vi "test.vi"() -> ()   [LabVIEW 2016, in "TCP文件传输系统.lvlib"]
uses:
  <vilib>/Utility/error.llb/whitespace.ctl
  <vilib>/Utility/sysdir.llb/System Directory Type.ctl
panel:
  out "枚举":T1(ring)
  in  "Version":string="版本升级文档.txt"
  out "TCP发送全局簇":T2
  out "文件传输的路径":path
  in  "Application":string="平台数据传输系统.exe"
  in  "远程端口或服务名称":u16=11234
  out "本机网络地址":string="192.168.1.250"
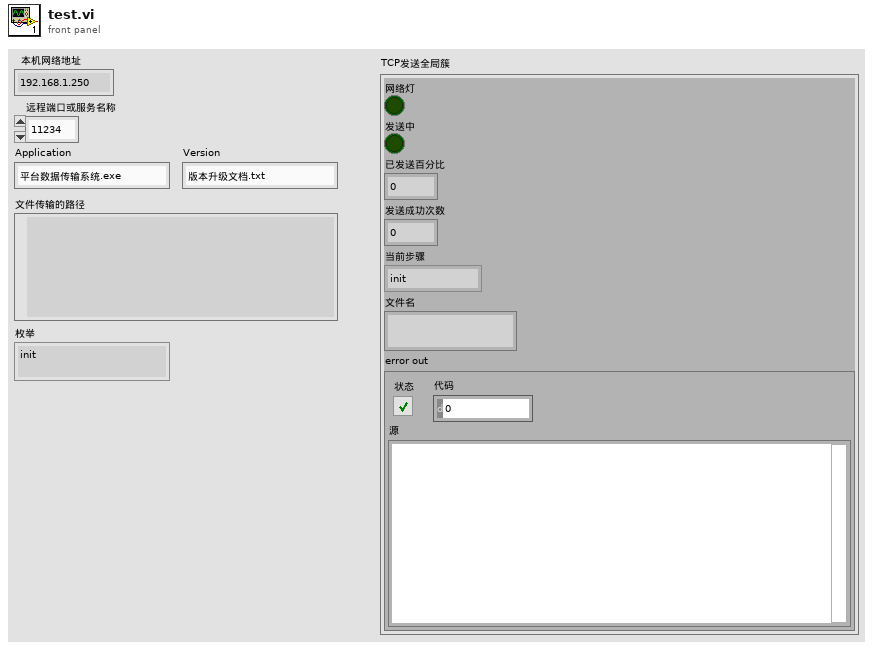
[diagram p1: front panel]
types:
  T1 = enum16{"init", "send version", "send version end", "send application", "send application end", "over"}
  T2 = cluster{"网络灯":bool, "发送中":bool, "已发送百分比":u8, "发送成功次数":dbl, "当前步骤":enum16{"init", "sendhead", "sendcontent", "sendsuccess", "over"}, "文件名":string, "error out":errorcluster}
  T3 = enum16{"Standard", "Buffered", "CRLF", "Immediate"}
  T4 = enum32{"Bad", "Idle", "Run top level", "Running"}
  T5 = typedef "whitespace.ctl" = u16
  T6 = typedef "System Directory Type.ctl" = i32
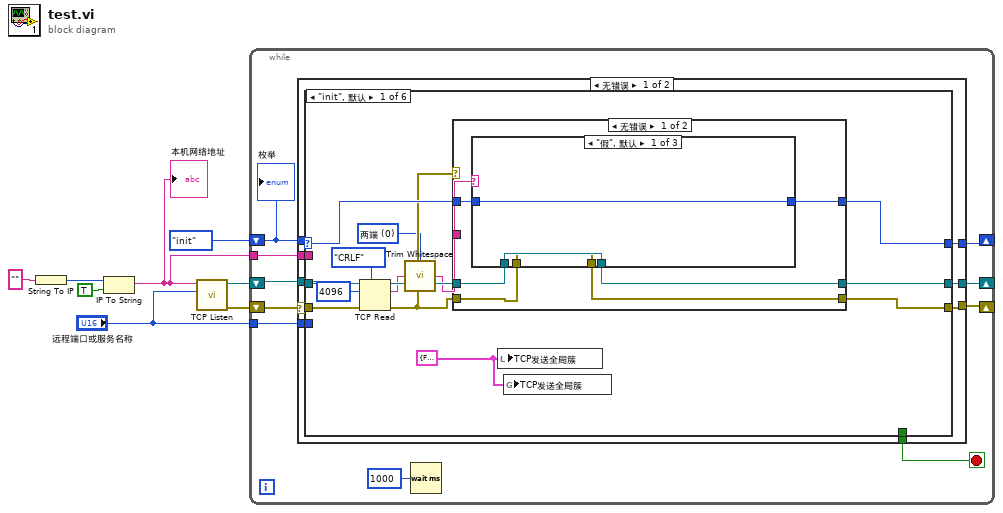
[diagram p0: block diagram]
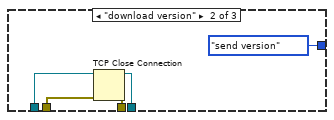
[diagram p2: hidden frame]
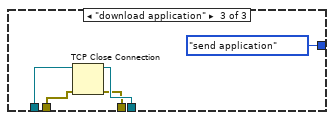
[diagram p3: hidden frame]
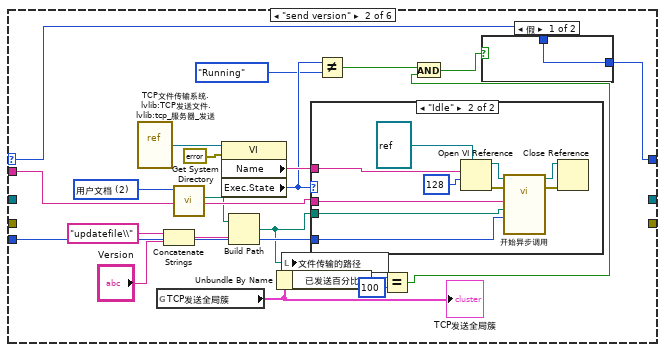
[diagram p5: hidden frame]
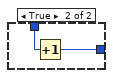
[diagram p6: hidden frame]
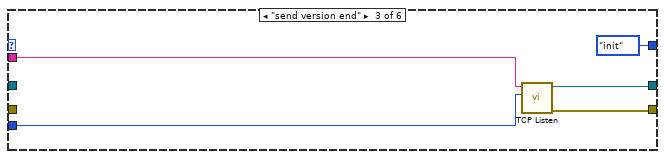
[diagram p8: hidden frame]
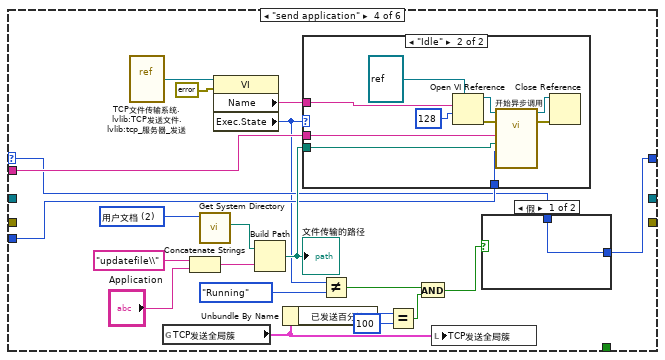
[diagram p9: hidden frame]
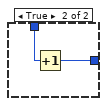
[diagram p10: hidden frame]
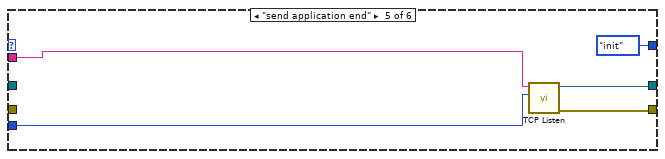
[diagram p12: hidden frame]
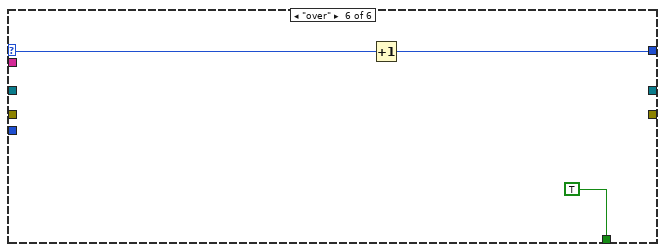
[diagram p13: hidden frame]
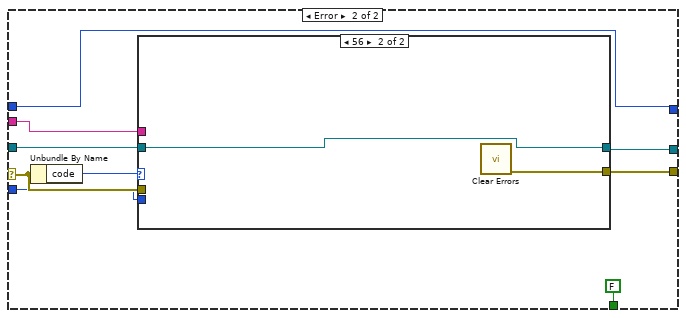
[diagram p14: hidden frame]
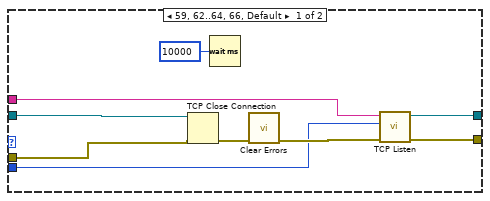
[diagram p15: hidden frame]
diagram:
  n1 = String To IP(1:"" ("名称")) -> (0:w5:u32)
  n2 = IP To String(1:TRUE ("句点符号？(F)"), 2:w5) -> (0:w1:string)
  "本机网络地址" <- w1
  n3 = call <vilib>:"TCP Listen.vi"("port"="远程端口或服务名称", "service name"=w1) -> ("error out"=w7:errorcluster, "connection ID"=w6:refnum<k5>)  [unwired: 5 in, 3 out]
  n4 = while {
    shift-right: [w17] -> _
    shift-left: T1."init" -> [w18]
    shift-right: [w12] -> _
    shift-left: w6 -> [w13]
    shift-right: [w11] -> _
    shift-left: w7 -> [w14]
    tunnel: w1 -> [w10]
    tunnel: "远程端口或服务名称" -> [w9]
    stop <- w16 stop-if-true
    n5 = case shown="无错误" w14 {
      selector: w14 -> [w23 w153]
      tunnel: w18 -> [w27 w149]
      tunnel: [w26 w149] -> w17
      tunnel: [w25 FALSE] -> w16
      tunnel: w13 -> [w24 w154]
      tunnel: [w22 w151] -> w12
      tunnel: [w21 w150] -> w11
      tunnel: w10 -> [w20 w147]
      tunnel: w9 -> [w19 w146]
      frame No Error {
        n6 = case shown="\"init\", 默认" w27 {
          selector: w27 -> [w40 w67 _ w113 _ w145]
          tunnel: [w39 w66 T1."init" w112 T1."init" w144] -> w26
          tunnel: [_ _ _ _ _ TRUE] -> w25
          tunnel: w24 -> [w33 _ _ _ _ _]
          tunnel: w23 -> [w41 _ _ _ _ _]
          tunnel: [w36 _ w100 _ w139 _] -> w22
          tunnel: [w35 _ w99 _ w138 _] -> w21
          tunnel: w20 -> [_ w82 w102 w115 w141 _]
          tunnel: w19 -> [_ w81 w101 w114 w140 _]
          frame "init", Default {
            w29 = T5 0 items=["两端", "字符串首端", "字符串末端"] ("location (both)")
            w34 = T2 {"网络灯"=FALSE, "发送中"=FALSE, "已发送百分比"=0, "发送成功次数"=0.0, "当前步骤"=enum."init", "文件名"="", "error out"={"status"=FALSE, "code"=0, "source"=""}} ("TCP发送全局簇")
            n7 = TCP Read(connection ID=w33, bytes to read=4096 ("读取的字节"), error in (no error)=w41, 7:T3."CRLF" ("模式（标准）")) -> (connection ID out=w38:refnum<k5>, data out=w30:string, error out=w37:errorcluster)  [unwired: 1 in]
            n8 = call <vilib>:"Trim Whitespace.vi"("string"=w30, "location (both)"=w29) -> ("trimmed string"=w28:string)
            n9 = case shown="无错误" w37 {
              tunnel: w28 -> [w48 _]
              tunnel: w40 -> [w47 w64]
              tunnel: [w46 w64] -> w39
              tunnel: w38 -> [w45 w63]
              tunnel: w37 -> [w44 w62]
              tunnel: [w43 w63] -> w36
              tunnel: [w42 w62] -> w35
              frame No Error {
                n10 = case shown="\"假\", 默认" w48 {
                  tunnel: w47 -> [w51 _ _]
                  tunnel: [w51 T1."send version" T1."send application"] -> w46
                  tunnel: w45 -> [w50 w55 w60]
                  tunnel: w44 -> [w49 w54 w59]
                  tunnel: [w50 w53 w58] -> w43
                  tunnel: [w49 w52 w57] -> w42
                  frame "假", Default {
                  }
                  frame "download version" {
                    n11 = TCP Close Connection(connection ID=w55, error in (no error)=w54) -> (connection ID out=w53:refnum<k5>, error out=w52:errorcluster)  [unwired: 1 in]
                  }
                  frame "download application" {
                    n12 = TCP Close Connection(connection ID=w60, error in (no error)=w59) -> (connection ID out=w58:refnum<k5>, error out=w57:errorcluster)  [unwired: 1 in]
                  }
                }
              }
              frame Error {
              }
            }
            n13 = local write "TCP发送全局簇"(w34) -> ()
            n14 = global write "全局变量1.vi" "TCP发送全局簇"(w34) -> ()
          }
          frame "send version" {
            w80 = T6 2 items=["用户目录"=0, "用户桌面"=1, "用户文档"=2, "用户应用程序数据"=3, "用户设置"=4, "用户临时目录"=5, "公共文档"=6, "公共应用程序数据"=7, "公共设置"=8, "公共缓存"=13, "系统核心库"=9, "系统安装库"=10, "应用程序文件"=11, "启动盘根目录"=12] ("system directory type")
            n15 = vi-ref "TCP文件传输系统.lvlib:TCP发送文件.lvlib:tcp_服务器_发送.vi"() -> (w83:refnum<vi>)
            n16 = global read "全局变量1.vi" "TCP发送全局簇"() -> (w73:T2)
            "TCP发送全局簇" <- w73
            n17 = Concatenate Strings("updatefile\\" ("condition"), "Version") -> (w77:string)
            n18 = call <vilib>:"Get System Directory.vi"("system directory type"=w80) -> ("system directory"=w79:path)  [unwired: 10 in]
            n19 = property class="VI"(reference=w83, error in=errorcluster {"status"=FALSE, "code"=0, "source"=""} ("错误输出")) -> ("Name"=w84:string, "Exec.State"=w75:T4)  [unwired: 2 out]
            n20 = Build Path(base path=w79, name or relative path=w77) -> (appended path=w65:path)
            n21 = Unbundle By Name(w73) -> ("已发送百分比"=w71:u8)
            n22 = local write "文件传输的路径"(w65) -> ()
            n23 = case shown="\"Idle\"" w75 {
              tunnel: w84 -> [_ w98]
              tunnel: w82 -> [_ w91]
              tunnel: w65 -> [_ w90]
              tunnel: w81 -> [_ w89]
              frame "Bad", Default {
              }
              frame "Idle" {
                n24 = Open VI Reference(type specifier VI Refnum (for type only)=refnum<vi> refnum, vi path=w98, options=128 ("选项")) -> (vi reference=w96:refnum<vi>, error out=w94:errorcluster)  [unwired: 3 in]
                n25 = call-by-ref "开始异步调用"(reference=w96, error in=w94, "远程端口或服务名称"=w89, "原文件路径（使用对话框）"=w90, "服务器网络地址"=w91) -> (reference out=w92:refnum<vi>, error out=w93:errorcluster)  [unwired: 9 in]
                n26 = Close Reference(reference=w92, error in (no error)=w93) -> ()  [unwired: 1 out]
              }
            }
            n27 = Not Equal?(x=w75, y=T4."Running") -> (x != y?=w72:bool)
            n28 = Equal?(x=w71, y=u8 100) -> (x = y?=w69:bool)
            n29 = And(x=w72, y=w69) -> (x .and. y?=w68:bool)
            n30 = case shown="假" w68 {
              tunnel: w67 -> [w86 w88]
              tunnel: [w86 w87] -> w66
              frame False {
              }
              frame True {
                n31 = Increment(x=w88) -> (x+1=w87:T1)
              }
            }
          }
          frame "send version end" {
            n32 = call <vilib>:"TCP Listen.vi"("port"=w101, "service name"=w102) -> ("error out"=w99:errorcluster, "connection ID"=w100:refnum<k5>)  [unwired: 5 in, 3 out]
          }
          frame "send application" {
            w116 = T6 2 items=["用户目录"=0, "用户桌面"=1, "用户文档"=2, "用户应用程序数据"=3, "用户设置"=4, "用户临时目录"=5, "公共文档"=6, "公共应用程序数据"=7, "公共设置"=8, "公共缓存"=13, "系统核心库"=9, "系统安装库"=10, "应用程序文件"=11, "启动盘根目录"=12] ("system directory type")
            n33 = vi-ref "TCP文件传输系统.lvlib:TCP发送文件.lvlib:tcp_服务器_发送.vi"() -> (w123:refnum<vi>)
            n34 = global read "全局变量1.vi" "TCP发送全局簇"() -> (w111:T2)
            n35 = Concatenate Strings("updatefile\\" ("condition"), "Application") -> (w119:string)
            n36 = call <vilib>:"Get System Directory.vi"("system directory type"=w116) -> ("system directory"=w117:path)  [unwired: 10 in]
            n37 = property class="VI"(reference=w123, error in=errorcluster {"status"=FALSE, "code"=0, "source"=""} ("错误输出")) -> ("Name"=w122:string, "Exec.State"=w104:T4)  [unwired: 2 out]
            n38 = Build Path(base path=w117, name or relative path=w119) -> (appended path=w124:path)
            "文件传输的路径" <- w124
            n39 = Unbundle By Name(w111) -> ("已发送百分比"=w106:u8)
            n40 = case shown="\"Idle\"" w104 {
              tunnel: w122 -> [_ w137]
              tunnel: w115 -> [_ w130]
              tunnel: w124 -> [_ w129]
              tunnel: w114 -> [_ w128]
              frame "Bad", Default {
              }
              frame "Idle" {
                n41 = Open VI Reference(type specifier VI Refnum (for type only)=refnum<vi> refnum, vi path=w137, options=128 ("选项")) -> (vi reference=w135:refnum<vi>, error out=w133:errorcluster)  [unwired: 3 in]
                n42 = call-by-ref "开始异步调用"(reference=w135, error in=w133, "远程端口或服务名称"=w128, "原文件路径（使用对话框）"=w129, "服务器网络地址"=w130) -> (reference out=w131:refnum<vi>, error out=w132:errorcluster)  [unwired: 9 in]
                n43 = Close Reference(reference=w131, error in (no error)=w132) -> ()  [unwired: 1 out]
              }
            }
            n44 = Not Equal?(x=w104, y=T4."Running") -> (x != y?=w109:bool)
            n45 = Equal?(x=w106, y=u8 100) -> (x = y?=w110:bool)
            n46 = And(x=w109, y=w110) -> (x .and. y?=w105:bool)
            n47 = local write "TCP发送全局簇"(w111) -> ()
            n48 = case shown="假" w105 {
              tunnel: w113 -> [w125 w127]
              tunnel: [w125 w126] -> w112
              frame False {
              }
              frame True {
                n49 = Increment(x=w127) -> (x+1=w126:T1)
              }
            }
          }
          frame "send application end" {
            n50 = call <vilib>:"TCP Listen.vi"("port"=w140, "service name"=w141) -> ("error out"=w138:errorcluster, "connection ID"=w139:refnum<k5>)  [unwired: 5 in, 3 out]
          }
          frame "over" {
            n51 = Increment(x=w145) -> (x+1=w144:T1)
          }
        }
      }
      frame Error {
        n52 = Unbundle By Name(w153) -> ("code"=w152:i32)
        n53 = case shown="56" w152 {
          tunnel: [w162 w164] -> w151
          tunnel: [w163 w165] -> w150
          tunnel: w154 -> [w159 w164]
          tunnel: w153 -> [w158 _]
          tunnel: w147 -> [w156 _]
          tunnel: w146 -> [w155 _]
          frame 59, 62..64, 66, Default {
            n54 = TCP Close Connection(connection ID=w159, error in (no error)=w158) -> (error out=w161:errorcluster)  [unwired: 1 in, 1 out]
            n55 = Wait (ms)(milliseconds to wait=u32 10000 ("等待时间（毫秒）")) -> ()  [unwired: 1 out]
            n56 = call <vilib>:"Clear Errors.vi"("error in (no error)"=w161) -> ("error out"=w160:errorcluster)  [unwired: 5 in, 1 out]
            n57 = call <vilib>:"TCP Listen.vi"("error in (no error)"=w160, "port"=w155, "service name"=w156) -> ("error out"=w163:errorcluster, "connection ID"=w162:refnum<k5>)  [unwired: 4 in, 3 out]
          }
          frame 56 {
            n58 = call <vilib>:"Clear Errors.vi"() -> ("error out"=w165:errorcluster)  [unwired: 6 in, 1 out]
          }
        }
      }
    }
    n59 = Wait (ms)(milliseconds to wait=u32 1000 ("等待时间（毫秒）")) -> ()  [unwired: 1 out]
    "枚举" <- w18
  }
